vi "Write Private Key.vi"(8 "error in (no error)":errorcluster, 10 "Private Key":path, 11 "SSL Server Context in":refnum<class "SSL Server Context.lvclass">) -> (0 "error out":errorcluster, 3 "SSL Server Context out":refnum<class "SSL Server Context.lvclass">)   [LabVIEW 2013, in "OpenSSL Socket.lvlib" / "SSL Server Context.lvclass"]
uses:
  SSL Server Context.lvclass
  SSL Server Context.lvclass/SSL Server Context.ctl
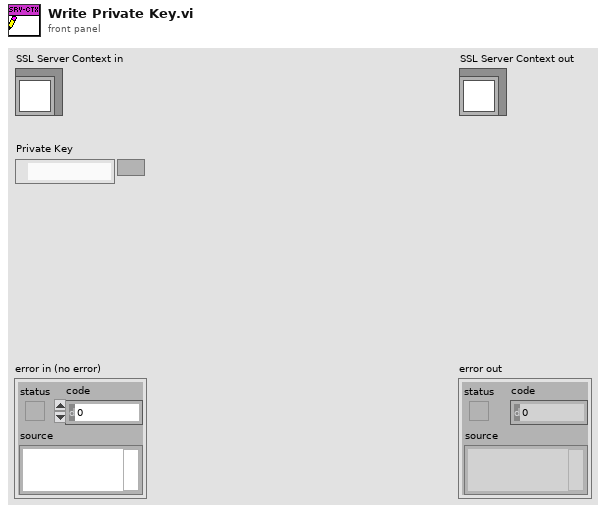
[diagram p1: front panel]
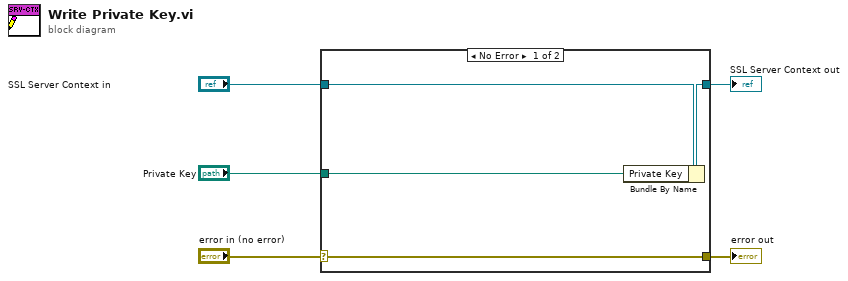
[diagram p0: block diagram]
diagram:
  n1 = case shown="No Error" "error in (no error)" {
    selector: "error in (no error)" -> [w9 w10]
    tunnel: [w9 w10] -> w4
    tunnel: [w7 w11] -> w2
    tunnel: "SSL Server Context in" -> [w8 w11]
    tunnel: "Private Key" -> [w6 _]
    frame No Error {
      n2 = Bundle By Name(cluster=w8, "Private Key"=w6) -> (w7:refnum<class "SSL Server Context.lvclass">)
    }
    frame Error {
    }
  }
  "error out" <- w4
  "SSL Server Context out" <- w2
